vi "Is Cell Valid.vi"(1 "Cell":cluster{"Row":i32, "Column":i32}) -> (0 "Valid?":bool)   [LabVIEW 2016, in "Excel.lvclass"]
uses:
  Excel.lvclass
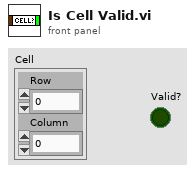
[diagram p1: front panel]
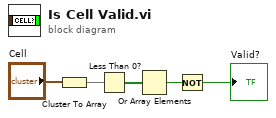
[diagram p0: block diagram]
diagram:
  n1 = Cluster To Array(cluster="Cell") -> (array=w4:i32[])
  n2 = Less Than 0?(x=w4) -> (x < 0?=w3:bool[])
  n3 = Or Array Elements(Boolean array=w3) -> (logical OR=w2:bool)
  n4 = Not(x=w2) -> (.not. x?=→"Valid?":bool)
